vi "Medicion de Tanque de Agua.vi"() -> ()   [LabVIEW 2019]
uses:
  <vilib>/Instr/_visa.llb/VISA Configure Serial Port (Instr).vi
panel:
  out "Histórico de la Temperatura":dbl(graph)
  out "Histórico del Nivel":dbl(graph)
  out "Temperatura":dbl(slide) scale=0.0..100.0 scale format="%#_g °C"
  out "Nivel":dbl(slide) scale=0.0..3.0 scale format="%#_g m"
  out "Alta Temperatura":bool
  out "Sobrecalentamiento":bool
  out "Nivel Alto":bool
  out "Desborde":bool
  out "Nivel Bajo":bool
  out "OK":bool
  in  "Alarma de Temperatura":dbl(knob)=100.0 scale=50.0..100.0
  in  "Nivel Bajo":dbl(knob)=0.5 scale=0.0..3.0
  in  "Advertencia de Temperatura":dbl(knob)=50.0 scale=25.0..75.0
  in  "Nivel Alto":dbl(knob)=2.0 scale=0.0..3.0
  in  "Paridad":enum16{"None", "Odd", "Even", "Mark", "Space"}(ring)
  in  "Tasa de Baudios":u32=9600
  in  "Recurso VISA":refnum<visa-resource-name>
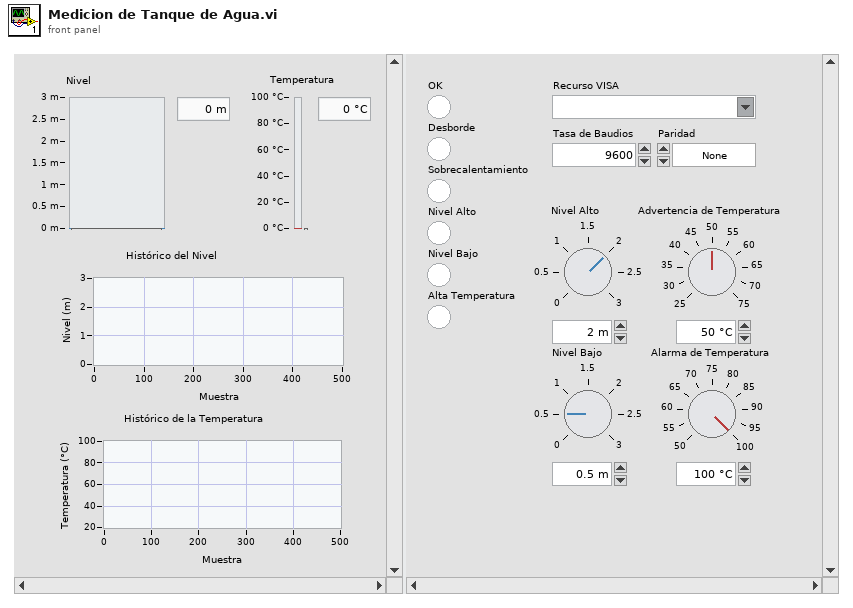
[diagram p1: front panel]
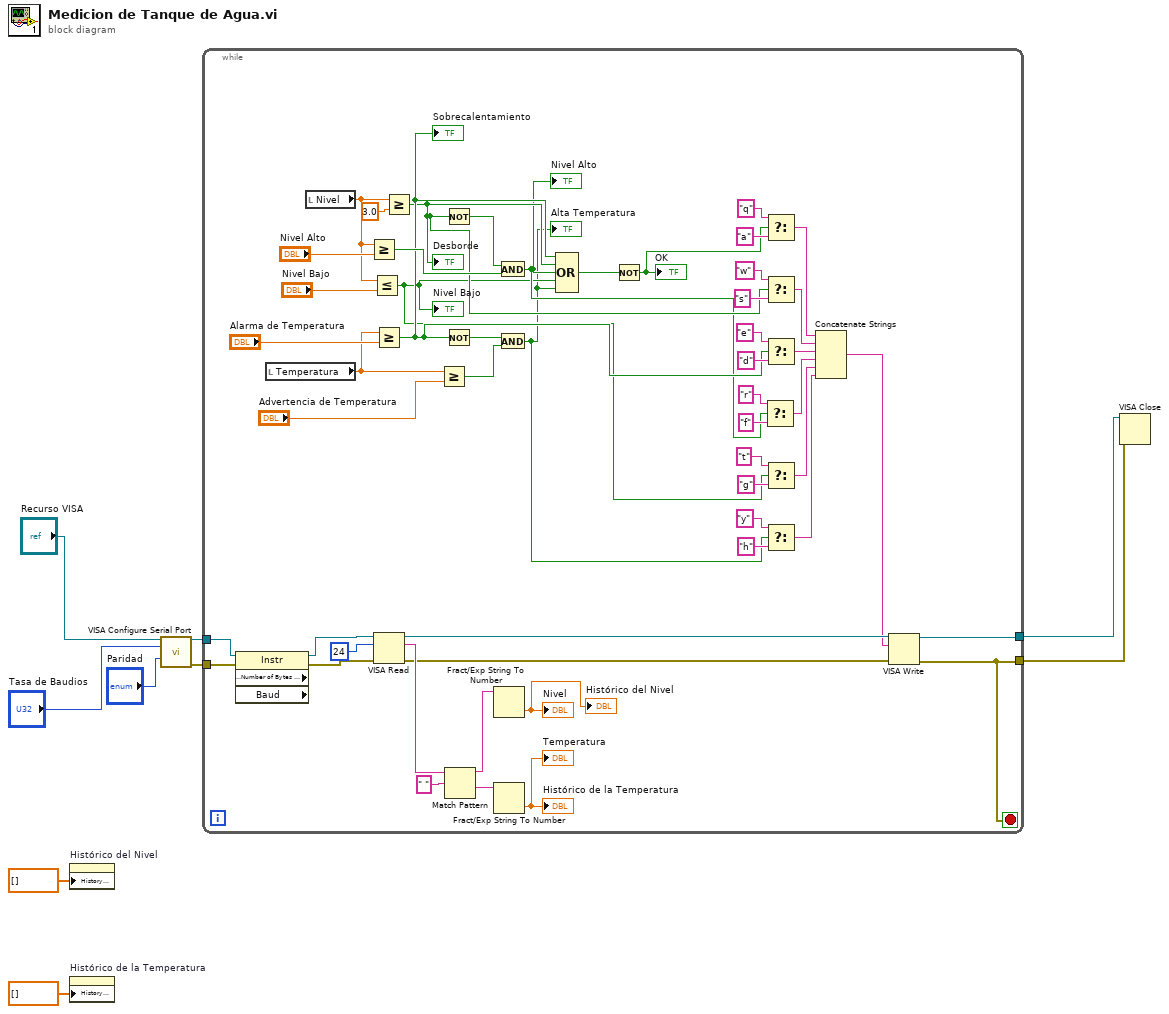
[diagram p0: block diagram]
diagram:
  n1 = property on="Histórico del Nivel" class="WFChart (strict)"("History Data"=dbl[] []) -> ()  [unwired: 2 in, 2 out]
  n2 = property on="Histórico de la Temperatura" class="WFChart (strict)"("History Data"=dbl[] []) -> ()  [unwired: 2 in, 2 out]
  n3 = call-poly "VISA Configure Serial Port"("VISA resource name"="Recurso VISA", "baud rate (9600)"="Tasa de Baudios", "parity (0:none)"="Paridad") -> ("VISA resource name out"=w6:refnum<visa-resource-name>, "error out"=w5:errorcluster)  [unwired: 11 in]
  n4 = while {
    tunnel: w6 -> [w58]
    tunnel: w5 -> [w57]
    tunnel: [w50] -> w2
    tunnel: [w10] -> w1
    stop <- w10 stop-if-true
    n5 = property class="Instr" props=["Serial Settings:Number of Bytes at Serial Port", "Baud"](reference=w58, error in=w57) -> (reference out=w61:refnum<visa-resource-name>, error out=w60:errorcluster)  [unwired: 2 out]
    n6 = local read "Temperatura"() -> (w20:dbl)
    n7 = local read "Nivel"() -> (w22:dbl)
    n8 = Greater Or Equal?(x=w22, y="Nivel Alto") -> (x >= y?=w25:bool)
    n9 = Less Or Equal?(x=w22, y="Nivel Bajo") -> (x <= y?=w13:bool)
    "Nivel Bajo" <- w13
    n10 = Greater Or Equal?(x=w20, y="Alarma de Temperatura") -> (x >= y?=w16:bool)
    "Sobrecalentamiento" <- w16
    n11 = VISA Read(VISA resource name=w61, byte count=u32 24, error in (no error)=w60) -> (VISA resource name out=w49:refnum<visa-resource-name>, read buffer=w51:string, error out=w48:errorcluster)  [unwired: 1 out]
    n12 = Greater Or Equal?(x=w22, y=3.0) -> (x >= y?=w15:bool)
    "Desborde" <- w15
    n13 = Greater Or Equal?(x=w20, y="Advertencia de Temperatura") -> (x >= y?=w19:bool)
    n14 = Not(x=w15) -> (.not. x?=w24:bool)
    n15 = Not(x=w16) -> (.not. x?=w18:bool)
    n16 = Match Pattern(string=w51, regular expression=" ") -> (before substring=w55:string, after substring=w54:string)  [unwired: 1 in, 2 out]
    n17 = Fract/Exp String To Number(string=w55) -> (number=→"Nivel" →"Histórico del Nivel":dbl)  [unwired: 3 in, 1 out]
    n18 = Fract/Exp String To Number(string=w54) -> (number=→"Temperatura" →"Histórico de la Temperatura":dbl)  [unwired: 3 in, 1 out]
    n19 = And(x=w24, y=w25) -> (x .and. y?=w14:bool)
    "Nivel Alto" <- w14
    n20 = And(x=w18, y=w19) -> (x .and. y?=w12:bool)
    "Alta Temperatura" <- w12
    n21 = Compound Arithmetic op=OR(w16, w15, w14, w13, w12) -> (w17:bool)
    n22 = Not(x=w17) -> (.not. x?=w11:bool)
    "OK" <- w11
    n23 = Select(t="r", s=w14, f="f") -> (s? t:f=w34:string)
    n24 = Select(t="q", s=w11, f="a") -> (s? t:f=w45:string)
    n25 = Select(t="w", s=w15, f="s") -> (s? t:f=w36:string)
    n26 = Select(t="e", s=w16, f="d") -> (s? t:f=w35:string)
    n27 = Select(t="t", s=w13, f="g") -> (s? t:f=w29:string)
    n28 = Select(t="y", s=w12, f="h") -> (s? t:f=w28:string)
    n29 = Concatenate Strings(w45, w36, w35, w34, w29, w28) -> (w47:string)
    n30 = VISA Write(VISA resource name=w49, write buffer=w47, error in (no error)=w48) -> (VISA resource name out=w50:refnum<visa-resource-name>, error out=w10:errorcluster)  [unwired: 1 out]
  }
  n31 = VISA Close(VISA resource name=w2, error in (no error)=w1) -> ()  [unwired: 1 out]
